vi "Gyro.vi"(10 "Reset":bool, 11 "Enum":enum16{"Start", "Run", "End"}(ring)) -> (3 "Angle":dbl)   [LabVIEW 2014]
uses:
  <vilib>/Rock Robotics/SystemInterfaces/Typedef/FPGA_TypedefAnalogModuleForGyro.ctl
  <vilib>/Rock Robotics/SystemInterfaces/AI/FPGA_AIGyroChannel.ctl
panel:
  out "Waveform Chart":dbl(graph)
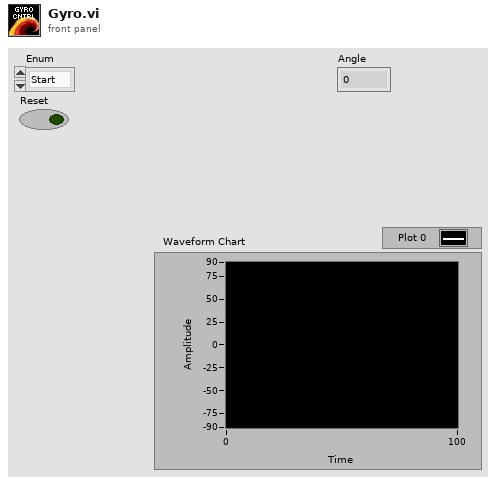
[diagram p1: front panel]
types:
  T1 = typedef "FPGA_AIGyroChannel.ctl" = enum8{"AI 1", "AI 2", "Invalid"}
  T2 = typedef "FPGA_TypedefAnalogModuleForGyro.ctl" = enum16{"Analog Module 1"}
  T3 = typedef "WPI_GyroDevRef.ctl" = cluster{"DevStatus":errorcluster, "Analog Module":T4, "Analog Channel":T5, "Offset":dbl, "Gain (VoltsPerDegree/Second)":dbl}
  T4 = typedef "FPGA_TypedefAnalogModule.ctl" = enum16{"Analog Module 1", "Analog Module 2"}
  T5 = typedef "FPGA_AIChannel.ctl" = enum8{"AI 1", "AI 2", "AI 3", "AI 4", "AI 5", "AI 6", "AI 7", "AI 8", "Invalid"}
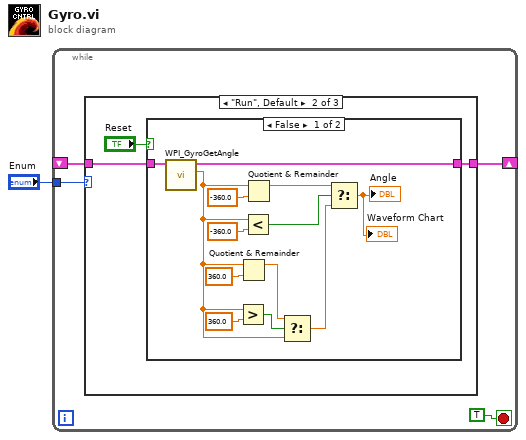
[diagram p0: block diagram]
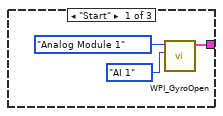
[diagram p2: hidden frame]
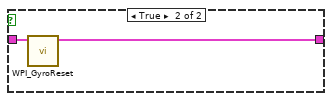
[diagram p3: hidden frame]
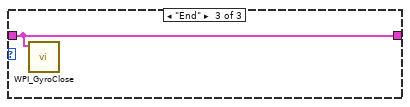
[diagram p4: hidden frame]
diagram:
  n1 = while {
    tunnel: "Enum" -> [w4]
    shift-right: [w2] -> _
    shift-left: _ -> [w3]
    stop <- TRUE stop-if-true
    n2 = case shown="\"Run\", Default" w4 {
      tunnel: w3 -> [_ w11 w27]
      tunnel: [w6 w10 w27] -> w2
      frame "Start" {
        n3 = call <vilib>:"WPI_GyroOpen.vi"("Analog Channel"=FPGA_AIGyroChannel."AI 1", "Analog Module (Module 1)"=FPGA_TypedefAnalogModuleForGyro."Analog Module 1") -> ("GyroDevRef"=w6:T3)  [unwired: 7 in, 2 out]
      }
      frame "Run", Default {
        n4 = case shown="False" "Reset" {
          tunnel: w11 -> [w24 w26]
          tunnel: [w23 w25] -> w10
          frame False {
            n5 = call <vilib>:"WPI_GyroGetAngle.vi"("GyroDevRef"=w24) -> ("Angle"=w14:dbl, "GyroDevRef"=w23:T3)  [unwired: 7 in, 2 out]
            n6 = Greater?(x=w14, y=360.0) -> (0:w20:bool)
            n7 = Quotient & Remainder(x=w14, y=360.0) -> (x-y*floor(x/y)=w13:dbl)  [unwired: 1 out]
            n8 = Less?(x=w14, y=-360.0) -> (x < y?=w19:bool)
            n9 = Quotient & Remainder(x=w14, y=-360.0) -> (x-y*floor(x/y)=w17:dbl)  [unwired: 1 out]
            n10 = Select(t=w13, s=w20, f=w14) -> (s? t:f=w18:dbl)
            n11 = Select(t=w17, s=w19, f=w18) -> (s? t:f=→"Angle" →"Waveform Chart":dbl)
          }
          frame True {
            n12 = call <vilib>:"WPI_GyroReset.vi"("GyroDevRef"=w26) -> ("GyroDevRef"=w25:T3)  [unwired: 9 in, 1 out]
          }
        }
      }
      frame "End" {
        n13 = call <vilib>:"WPI_GyroClose.vi"("GyroDevRef"=w27) -> ()  [unwired: 10 in, 1 out]
      }
    }
  }
